vi "Probability Bar.vi"(7 "QuWire in":refnum<class "QuWire.lvclass">) -> ()   [LabVIEW 2020]
uses:
  QuSim/QuWire/QuWire.lvclass
panel:
  out "Probability Bar Graph":cluster{i32[], dbl[]}(graph)
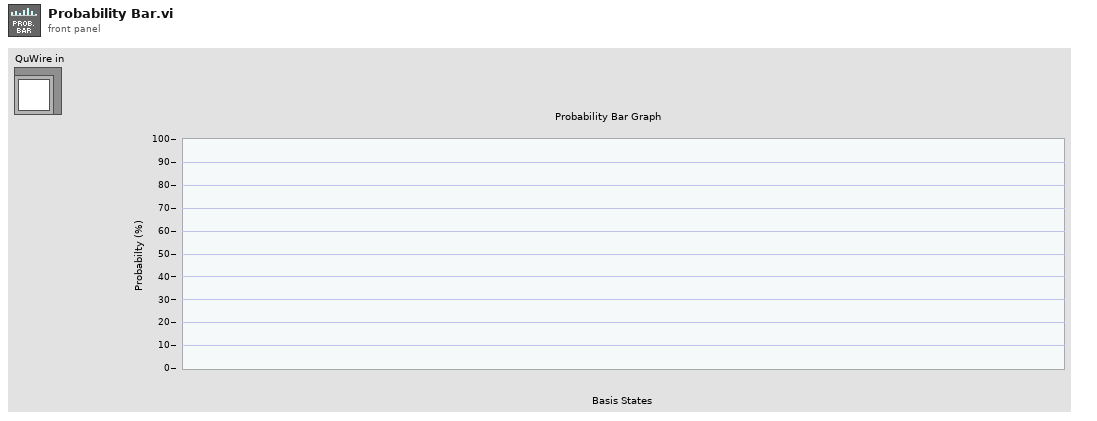
[diagram p1: front panel]
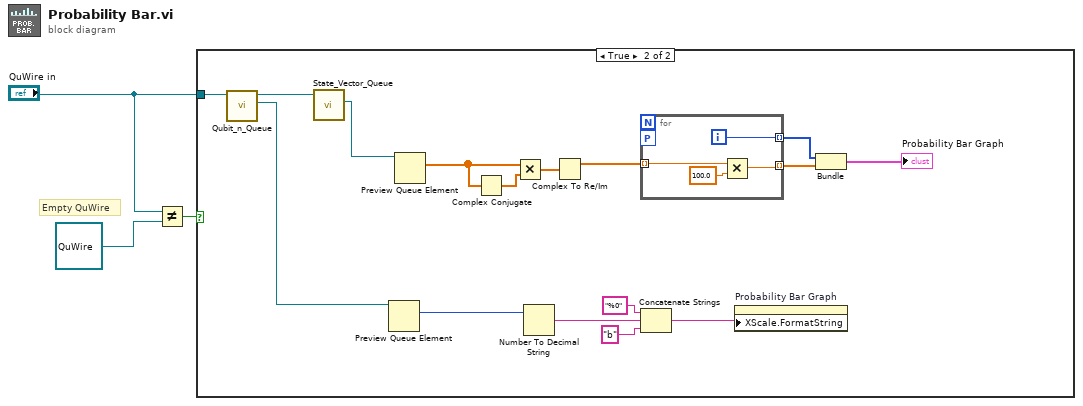
[diagram p0: block diagram]
diagram:
  # "Empty QuWire"
  n1 = Not Equal?(x="QuWire in", y=refnum<class "QuWire.lvclass"> refnum ("QuWire in")) -> (x != y?=w2:bool)
  n2 = case shown="True" w2 {
    tunnel: "QuWire in" -> [_ w14]
    frame False {
    }
    frame True {
      n3 = call "Qubit_n_Queue.vi"("QuWire in"=w14) -> ("Qubit n"=w13:refnum<queue>, "QuWire out"=w15:refnum<class "QuWire.lvclass">)  [unwired: 8 in, 1 out]
      n4 = call "State_Vector_Queue.vi"("QuWire in"=w15) -> ("State Vector Queue"=w19:refnum<queue>)  [unwired: 8 in, 2 out]
      n5 = Preview Queue Element(queue=w13) -> (element=w9:i32)  [unwired: 2 in, 3 out]
      n6 = Preview Queue Element(queue=w19) -> (element=w17:cdb[])  [unwired: 2 in, 3 out]
      n7 = Complex Conjugate(1:w17) -> (0:w18:cdb[])
      n8 = Multiply(x=w17, y=w18) -> (x*y=w16:cdb[])
      n9 = Number To Decimal String(number=w9) -> (decimal integer string=w10:string)  [unwired: 1 in]
      n10 = Complex To Re/Im(x + iy=w16) -> (x=w4:dbl[])  [unwired: 1 out]
      n11 = for {
        tunnel: w4 -> [w21] mode=indexing
        workers-P: _ -> [_]
        tunnel: [w23] -> w7 mode=indexing
        tunnel: [w20] -> w6 mode=indexing
        i -> [w23]
        n12 = Multiply(x=w21, y=100.0) -> (x*y=w20:dbl)
      }
      n13 = Concatenate Strings("%0" ("string"), w10, "b" ("string")) -> (w5:string)
      n14 = property on="Probability Bar Graph" class="XYGraph (strict)"("XScale.FormatString"=w5) -> ()  [unwired: 2 in, 2 out]
      n15 = Bundle(w7, w6) -> (→"Probability Bar Graph":cluster{i32[], dbl[]})  [unwired: 1 in]
    }
  }
